vi "d1000 set command pos.vi"(10 "Pos":dbl, 11 "axis":i16) -> (3 "function return":u32)   [LabVIEW 2019, in "Dmc1000.lvlib"]
doc: "DMC1000_API DWORD WINAPI d1000_set_command_pos(short axis,double Pos);"
uses:
  Dmc1000.lvlib
  Dmc1000.dll
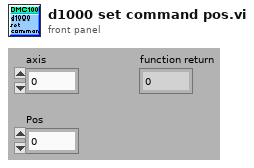
[diagram p1: front panel]
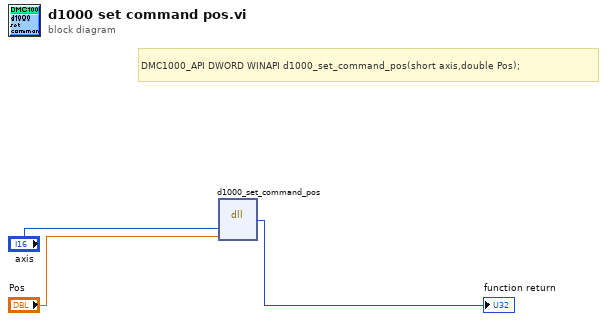
[diagram p0: block diagram]
diagram:
  # "DMC1000_API DWORD WINAPI d1000_set_command_pos(short axis,double Pos);"
  n1 = dll-call lib="C:/Users/VIC/Desktop/Standar Program/System/LLB/DMC1000B/Dmc1000.*" fn="d1000_set_command_pos"("axis"="axis", "Pos"="Pos") -> (→"function return":u32)  [unwired: 5 in, 2 out]
